vi "Shared Binary Version (DNN).vi"(8 "error in (no error)":errorcluster) -> (0 "error out":errorcluster, 3 "Version":string)   [LabVIEW 2020, in "feature_detection.lvlib"]
doc: "Get the version of the shared binary file for this component."
uses:
  feature_detection.lvlib
  common/common.lvlib
  common/bin/gartoolkit_dnn_32-1.dll
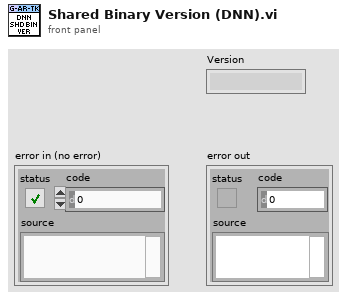
[diagram p1: front panel]
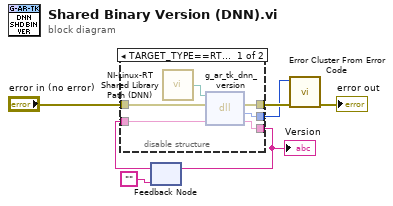
[diagram p0: block diagram]
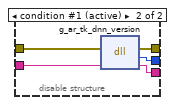
[diagram p2: hidden frame]
diagram:
  n1 = feedback #1("") -> (w5:string)
  n2 = disable-structure "Conditional Disable Structure" shown="TARGET_TYPE==RT&&OS==Linux" {
    disable-tunnel: [w10 w18] -> w3
    disable-tunnel: [w12 w17] -> w6
    disable-tunnel: w5 -> [w13 w16]
    disable-tunnel: [w11 w15] -> w4
    disable-tunnel: "error in (no error)" -> [w8 w14]
    frame condition #0 {
      n3 = call "NI-Linux-RT Shared Library Path (DNN).vi"() -> ("Path"=w9:path)
      n4 = dll-call lib="?" fn="g_ar_tk_dnn_version" ("g_ar_toolkit.*.*:g_ar_tk_capture_context_create")(path in=w9, error in=w8, "version"=w13) -> (error out=w11:errorcluster, "return type"=w10:i32, "version"=w12:string)  [unwired: 1 in, 1 out]
    }
    frame condition #1 (active) {
      n5 = dll-call lib="C:/serenial/lib/g-augmented-reality-toolkit/LabVIEW/common/bin/gartoolkit_dnn_*-1.*" fn="g_ar_tk_dnn_version" ("g_ar_toolkit.*.*:g_ar_tk_capture_context_create")(error in=w14, "version"=w16) -> (error out=w15:errorcluster, "return type"=w18:i32, "version"=w17:string)  [unwired: 2 in, 1 out]
    }
  }
  "Version" <- w6
  n6 = feedback-in #1(w6) -> ()
  n7 = call <vilib>:"Error Cluster From Error Code.vi"("error in (no error)"=w4, "error code (0)"=w3) -> ("error out"=→"error out":errorcluster)  [unwired: 7 in]
